vi "PH_Init.vi"(0 "MAXDEV":i32=8, 11 "error in (no error)":errorcluster) -> (4 "Library Version":string="2.1", 6 "Device List":T1(array[cluster]), 15 "error out":errorcluster)   [LabVIEW 8.6]
doc: "Prepare PicoHarp 300 for T3R-Measurement"
uses:
  MT Scan/SubVIs/PHLib.dll
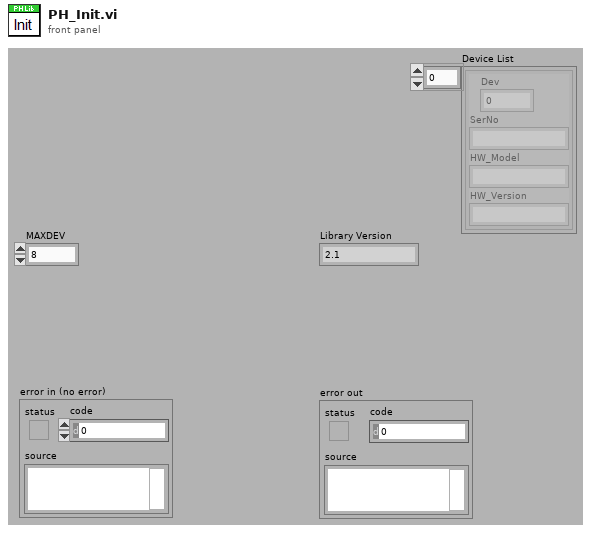
[diagram p1: front panel]
types:
  T1 = cluster{"Dev":i32, "SerNo":string, "HW_Model":string, "HW_Version":string}[]
  T2 = cluster{"Dev":i32, "SerNo":string, "HW_Model":string, "HW_Version":string}
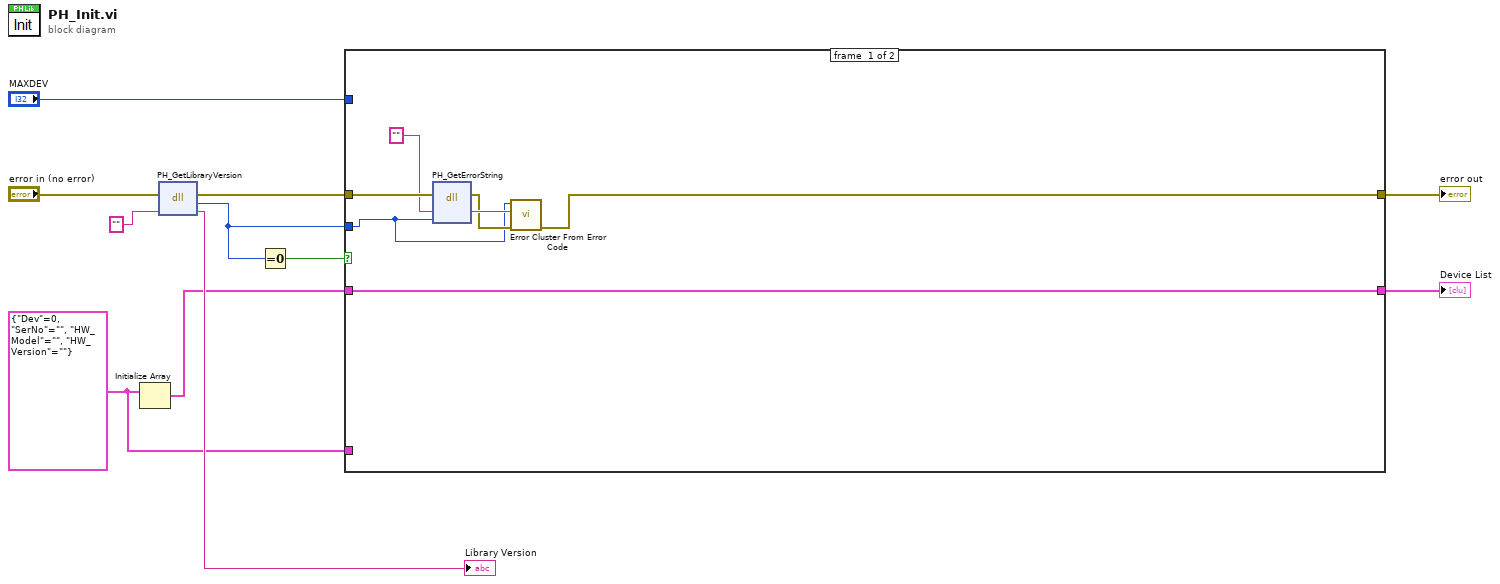
[diagram p0: block diagram]
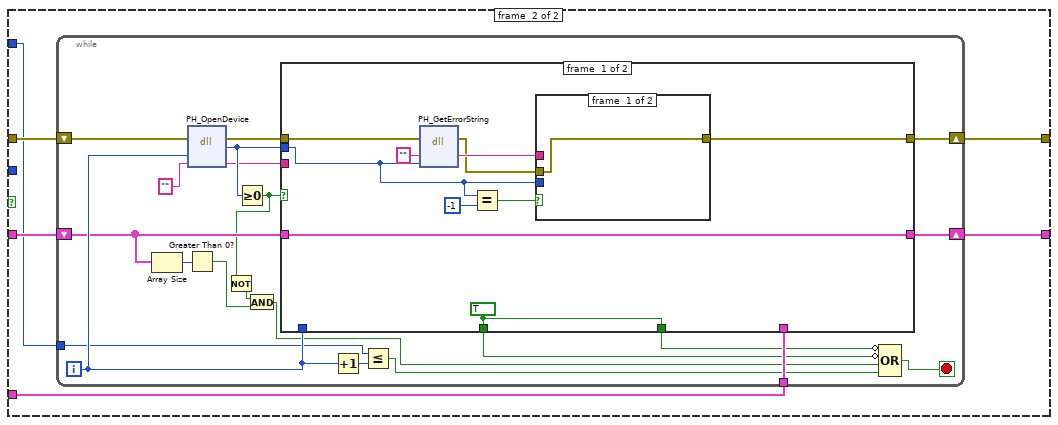
[diagram p2: hidden frame]
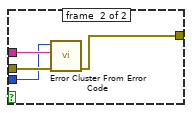
[diagram p3: hidden frame]
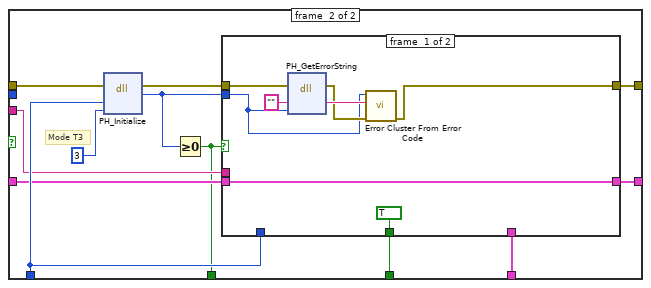
[diagram p4: hidden frame]
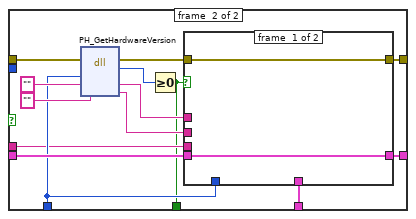
[diagram p5: hidden frame]
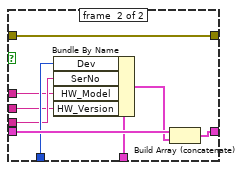
[diagram p6: hidden frame]
diagram:
  w2 = T2 {"Dev"=0, "SerNo"="", "HW_Model"="", "HW_Version"=""}
  n1 = Initialize Array(w2) -> (w3:T1)  [unwired: 1 in]
  n2 = dll-call lib="C:/LabVIEW Programs/MT Scan/SubVIs/PHLib.dll" fn="PH_GetLibraryVersion"(error in="error in (no error)", "vers"="") -> (error out=w8:errorcluster, "return type"=w4:i32, "vers"=→"Library Version":string)  [unwired: 2 in, 1 out]
  n3 = Equal To 0?(x=w4) -> (x = 0?=w5:bool)
  n4 = case shown="True" w5 {
    tunnel: w8 -> [w18 w24]
    tunnel: "MAXDEV" -> [_ w19]
    tunnel: [w15 w23] -> w6
    tunnel: w4 -> [w12 _]
    tunnel: w3 -> [w13 w22]
    tunnel: w2 -> [_ w21]
    tunnel: [w13 w20] -> w1
    frame #0 {
      n5 = dll-call lib="C:/LabVIEW Programs/MT Scan/SubVIs/PHLib.dll" fn="PH_GetErrorString"(error in=w18, "errstring"="", "errcode"=w12) -> (error out=w16:errorcluster, "errstring"=w17:string)  [unwired: 4 in, 1 out]
      n6 = call <vilib>:"Error Cluster From Error Code.vi"("error in (no error)"=w16, "error message (\"\")"=w17, "error code (0)"=w12) -> ("error out"=w15:errorcluster)  [unwired: 6 in]
    }
    frame #1 {
      n7 = while {
        shift-right: [w41] -> w23
        shift-left: w24 -> [w45]
        shift-right: [w39] -> w20
        shift-left: w22 -> [w30]
        tunnel: w21 -> [w38]
        tunnel: w19 -> [w34]
        i -> [w36]
        stop <- w37 stop-if-true
        n8 = Array Size(array=w30) -> (size(s)=w29:i32)
        n9 = Greater Than 0?(x=w29) -> (x > 0?=w28:bool)
        n10 = dll-call lib="C:/LabVIEW Programs/MT Scan/SubVIs/PHLib.dll" fn="PH_OpenDevice"(error in=w45, "devidx"=w36, "serial"="" ("vers")) -> (error out=w43:errorcluster, "return type"=w42:i32, "serial"=w40:string)  [unwired: 3 in, 1 out]
        n11 = Greater Or Equal To 0?(x=w42) -> (x >= 0?=w26:bool)
        n12 = Not(x=w26) -> (.not. x?=w27:bool)
        n13 = And(x=w27, y=w28) -> (x .and. y?=w25:bool)
        n14 = case shown="False" w26 {
          tunnel: w43 -> [w53 w72]
          tunnel: w36 -> [_ w67]
          tunnel: w42 -> [w48 _]
          tunnel: [w52 w68] -> w41
          tunnel: w40 -> [_ w63]
          tunnel: w30 -> [w50 w66]
          tunnel: [w50 w65] -> w39
          tunnel: w38 -> [_ w64]
          tunnel: [w49 w62] -> w32
          tunnel: [w49 w61] -> w31
          frame #0 {
            w49 = TRUE
            n15 = dll-call lib="C:/LabVIEW Programs/MT Scan/SubVIs/PHLib.dll" fn="PH_GetErrorString"(error in=w53, "errstring"="", "errcode"=w48) -> (error out=w54:errorcluster, "errstring"=w55:string)  [unwired: 4 in, 1 out]
            n16 = Equal?(x=w48, y=-1) -> (x = y?=w46:bool)
            n17 = case shown="False" w46 {
              tunnel: w55 -> [_ w60]
              tunnel: w54 -> [w56 w59]
              tunnel: [w56 w58] -> w52
              tunnel: w48 -> [_ w57]
              frame #0 {
              }
              frame #1 {
                n18 = call <vilib>:"Error Cluster From Error Code.vi"("error in (no error)"=w59, "error message (\"\")"=w60, "error code (0)"=w57) -> ("error out"=w58:errorcluster)  [unwired: 6 in]
              }
            }
          }
          frame #1 {
            # "Mode T3"
            n19 = dll-call lib="C:/LabVIEW Programs/MT Scan/SubVIs/PHLib.dll" fn="PH_Initialize"(error in=w72, "devidx"=w67, "mode"=3) -> (error out=w70:errorcluster, "return type"=w69:i32)  [unwired: 4 in, 1 out]
            n20 = Greater Or Equal To 0?(x=w69) -> (x >= 0?=w62:bool)
            n21 = case shown="True" w62 {
              tunnel: w70 -> [w78 w94]
              tunnel: w69 -> [w74 _]
              tunnel: [w77 w91] -> w68
              tunnel: w67 -> [_ w85]
              tunnel: w66 -> [w75 w88]
              tunnel: [w75 w87] -> w65
              tunnel: w64 -> [_ w86]
              tunnel: w63 -> [_ w84]
              tunnel: [TRUE w81] -> w61
              frame #0 {
                n22 = dll-call lib="C:/LabVIEW Programs/MT Scan/SubVIs/PHLib.dll" fn="PH_GetErrorString"(error in=w78, "errstring"="", "errcode"=w74) -> (error out=w79:errorcluster, "errstring"=w80:string)  [unwired: 4 in, 1 out]
                n23 = call <vilib>:"Error Cluster From Error Code.vi"("error in (no error)"=w79, "error message (\"\")"=w80, "error code (0)"=w74) -> ("error out"=w77:errorcluster)  [unwired: 6 in]
              }
              frame #1 {
                n24 = dll-call lib="C:/LabVIEW Programs/MT Scan/SubVIs/PHLib.dll" fn="PH_GetHardwareVersion"(error in=w94, "devidx"=w85, "model"="", "version"="") -> (error out=w92:errorcluster, "return type"=w93:i32, "model"=w82:string, "version"=w83:string)  [unwired: 3 in, 1 out]
                n25 = Greater Or Equal To 0?(x=w93) -> (x >= 0?=w81:bool)
                n26 = case shown="True" w81 {
                  tunnel: w92 -> [w96 w105]
                  tunnel: [w96 w105] -> w91
                  tunnel: w88 -> [w95 w104]
                  tunnel: [w95 w103] -> w87
                  tunnel: w86 -> [_ w102]
                  tunnel: w85 -> [_ w100]
                  tunnel: w84 -> [_ w99]
                  tunnel: w83 -> [_ w98]
                  tunnel: w82 -> [_ w97]
                  frame #0 {
                  }
                  frame #1 {
                    n27 = Bundle By Name(cluster=w102, "Dev"=w100, "SerNo"=w99, "HW_Model"=w97, "HW_Version"=w98) -> (w101:T2)
                    n28 = Build Array (concatenate)(w104, w101) -> (w103:T1)
                  }
                }
              }
            }
          }
        }
        n29 = Increment(x=w36) -> (x+1=w35:i32)
        n30 = Less Or Equal?(x=w34, y=w35) -> (x <= y?=w33:bool)
        n31 = Compound Arithmetic op=OR(invert w31, invert w32, w25, w33) -> (w37:bool)
      }
    }
  }
  "error out" <- w6
  "Device List" <- w1
